vi "AO Wave.vi"() -> ()   [LabVIEW 2016]
panel:
  out "error out":errorcluster caption="错误输出"
  out "波形图":dbl[](graph)
  in  "WaveSampleRate(pts/s)":u32=100000
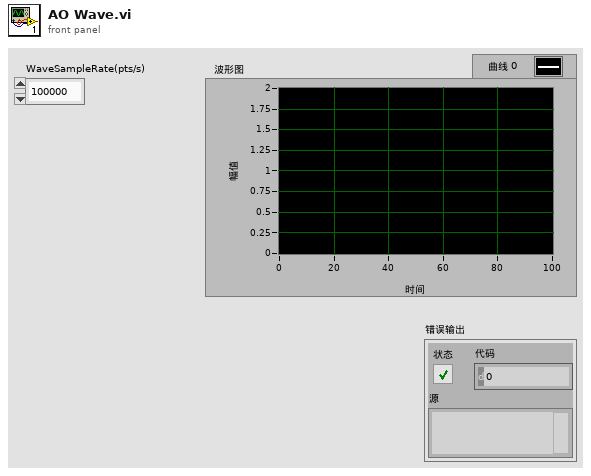
[diagram p1: front panel]
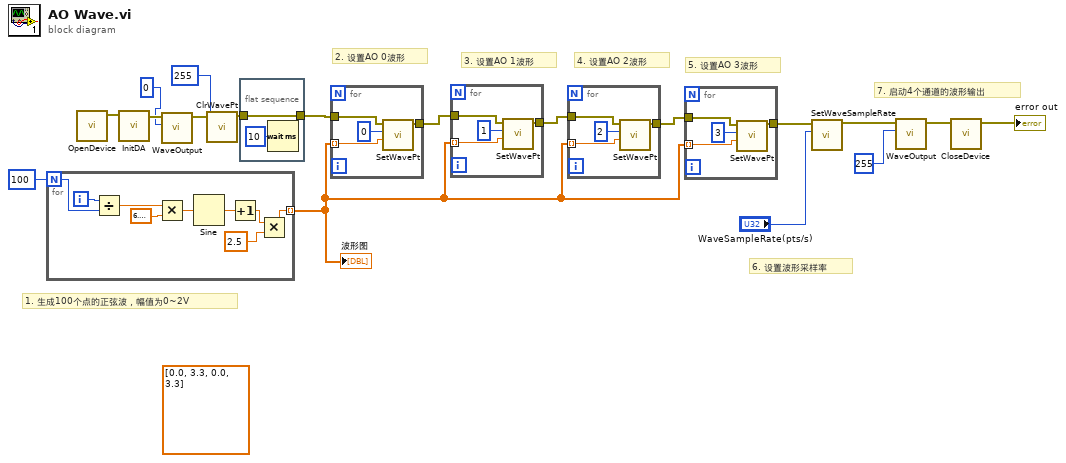
[diagram p0: block diagram]
diagram:
  (unwired) dbl[] [0.0, 3.3, 0.0, 3.3]
  # "7. 启动4个通道的波形输出"
  # "6. 设置波形采样率"
  # "5. 设置AO 3波形"
  # "4. 设置AO 2波形"
  # "3. 设置AO 1波形"
  # "2. 设置AO 0波形"
  # "1. 生成100个点的正弦波，幅值为0~2V"
  n1 = for {
    N: 100 -> [w26]
    tunnel: [w19] -> w2 mode=indexing
    i -> [w27]
    n2 = Divide(x=w27, y=w26) -> (x/y=w25:dbl)
    n3 = Multiply(x=w25, y=6.283185307179586) -> (x*y=w23:dbl)
    n4 = Sine(x=w23) -> (sin(x)=w22:dbl)
    n5 = Increment(x=w22) -> (x+1=w21:dbl)
    n6 = Multiply(x=w21, y=2.5) -> (x*y=w19:dbl)
  }
  "波形图" <- w2
  n7 = call "OpenDevice.vi"() -> ("error out"=w17:errorcluster)  [unwired: 11 in]
  n8 = call "InitDA.vi"("error in"=w17) -> ("error out"=w10:errorcluster)  [unwired: 10 in]
  n9 = call "WaveOutput.vi"("DANum"=u8 0, "error in"=w10) -> ("error out"=w9:errorcluster)  [unwired: 9 in]
  n10 = call "ClrWavePt.vi"("DaNum"=u8 255, "error in"=w9) -> ("error out"=w5:errorcluster)  [unwired: 9 in]
  n11 = flat-sequence {
    tunnel: [w29] -> w6
    tunnel: w5 -> [w29]
    frame #0 {
      n12 = Wait (ms)(milliseconds to wait=u32 10 ("等待时间（毫秒）")) -> ()  [unwired: 1 out]
    }
  }
  n13 = for {
    tunnel: w6 -> [w33]
    tunnel: w2 -> [w32] mode=indexing
    tunnel: [w30] -> w16
    n14 = call "SetWavePt.vi"("Voltage"=w32, "DaNum"=u8 0, "error in"=w33) -> ("error out"=w30:errorcluster)  [unwired: 8 in]
  }
  n15 = for {
    tunnel: w16 -> [w37]
    tunnel: w2 -> [w36] mode=indexing
    tunnel: [w34] -> w15
    n16 = call "SetWavePt.vi"("Voltage"=w36, "DaNum"=u8 1, "error in"=w37) -> ("error out"=w34:errorcluster)  [unwired: 8 in]
  }
  n17 = for {
    tunnel: w15 -> [w41]
    tunnel: w2 -> [w40] mode=indexing
    tunnel: [w38] -> w14
    n18 = call "SetWavePt.vi"("Voltage"=w40, "DaNum"=u8 2, "error in"=w41) -> ("error out"=w38:errorcluster)  [unwired: 8 in]
  }
  n19 = for {
    tunnel: w14 -> [w45]
    tunnel: w2 -> [w44] mode=indexing
    tunnel: [w42] -> w1
    n20 = call "SetWavePt.vi"("Voltage"=w44, "DaNum"=u8 3, "error in"=w45) -> ("error out"=w42:errorcluster)  [unwired: 8 in]
  }
  n21 = call "SetWaveSampleRate.vi"("WaveSampleRate(pts/s)"="WaveSampleRate(pts/s)", "error in"=w1) -> ("error out"=w12:errorcluster)  [unwired: 9 in]
  n22 = call "WaveOutput.vi"("DANum"=u8 255, "error in"=w12) -> ("error out"=w4:errorcluster)  [unwired: 9 in]
  n23 = call "CloseDevice.vi"("error in"=w4) -> ("error out"=→"error out":errorcluster)  [unwired: 10 in]
